vi "Main.vi"(7 "sweep rate, /min":dbl=0.2, 8 "sweep to:":dbl=-0.5, 9 "sweep":T6(radio)=enum."time_sweep") -> ()   [LabVIEW 2017] (continued)
                            n1353 = property on="data" class="Arr (strict)"("Value"=w1722) -> ()  [unwired: 2 in, 2 out]
                          }
                          frame #42 {
                            # "check if current \non 2461 SouceMeter\nis to be measured"
                            n1354 = property on="data" class="Arr (strict)"() -> ("Value"=w1730:dbl[])  [unwired: 2 in, 2 out]
                            n1355 = property on="iTC_Sample_T" class="Bool (strict)"() -> ("Value"=w1729:bool)  [unwired: 2 in, 2 out]
                            n1356 = case shown="True" w1729 {
                              tunnel: w1730 -> [w1732 w1737]
                              tunnel: [w1732 w1736] -> w1731
                              frame False {
                                # "we are not measuring 2461, voltage (2461_meas_v)"
                              }
                              frame True {
                                # "we are  measuring 2461, voltage (2461_meas_v)"
                                n1357 = property on="iTC_addr_sweep" class="VISAName"() -> ("Value"=w1735:refnum<visa-resource-name>)  [unwired: 2 in, 2 out]
                                n1358 = call "iTCread.vi"("VISA resource name"=w1735, "iTCreadCtrl"=iTCreadCtrl."Sample Temp") -> ("number"=w1733:dbl)  [unwired: 5 in, 3 out]
                                n1359 = Build Array (concatenate)(w1737, w1733) -> (w1736:dbl[])
                              }
                            }
                            n1360 = property on="data" class="Arr (strict)"("Value"=w1731) -> ()  [unwired: 2 in, 2 out]
                          }
                          frame #43 {
                            # "check if current \non 2461 SouceMeter\nis to be measured"
                            n1361 = property on="data" class="Arr (strict)"() -> ("Value"=w1739:dbl[])  [unwired: 2 in, 2 out]
                            n1362 = property on="VTI_T" class="Bool (strict)"() -> ("Value"=w1738:bool)  [unwired: 2 in, 2 out]
                            n1363 = case shown="True" w1738 {
                              tunnel: w1739 -> [w1741 w1746]
                              tunnel: [w1741 w1745] -> w1740
                              frame False {
                                # "we are not measuring 2461, voltage (2461_meas_v)"
                              }
                              frame True {
                                # "we are  measuring 2461, voltage (2461_meas_v)"
                                n1364 = property on="iTC_addr_sweep" class="VISAName"() -> ("Value"=w1744:refnum<visa-resource-name>)  [unwired: 2 in, 2 out]
                                n1365 = call "iTCread.vi"("VISA resource name"=w1744, "iTCreadCtrl"=iTCreadCtrl."VTI Temp") -> ("number"=w1742:dbl)  [unwired: 5 in, 3 out]
                                n1366 = Build Array (concatenate)(w1746, w1742) -> (w1745:dbl[])
                              }
                            }
                            n1367 = property on="data" class="Arr (strict)"("Value"=w1740) -> ()  [unwired: 2 in, 2 out]
                          }
                          frame #44 {
                            # "check if current \non 2461 SouceMeter\nis to be measured"
                            n1368 = property on="data" class="Arr (strict)"() -> ("Value"=w1748:dbl[])  [unwired: 2 in, 2 out]
                            n1369 = property on="PT1_T" class="Bool (strict)"() -> ("Value"=w1747:bool)  [unwired: 2 in, 2 out]
                            n1370 = case shown="True" w1747 {
                              tunnel: w1748 -> [w1750 w1755]
                              tunnel: [w1750 w1754] -> w1749
                              frame False {
                                # "we are not measuring 2461, voltage (2461_meas_v)"
                              }
                              frame True {
                                # "we are  measuring 2461, voltage (2461_meas_v)"
                                n1371 = property on="iTC_addr_sweep" class="VISAName"() -> ("Value"=w1753:refnum<visa-resource-name>)  [unwired: 2 in, 2 out]
                                n1372 = call "iTCread.vi"("VISA resource name"=w1753, "iTCreadCtrl"=iTCreadCtrl."PT1 Temp") -> ("number"=w1751:dbl)  [unwired: 5 in, 3 out]
                                n1373 = Build Array (concatenate)(w1755, w1751) -> (w1754:dbl[])
                              }
                            }
                            n1374 = property on="data" class="Arr (strict)"("Value"=w1749) -> ()  [unwired: 2 in, 2 out]
                          }
                          frame #45 {
                            # "check if current \non 2461 SouceMeter\nis to be measured"
                            n1375 = property on="data" class="Arr (strict)"() -> ("Value"=w1757:dbl[])  [unwired: 2 in, 2 out]
                            n1376 = property on="PT2_T" class="Bool (strict)"() -> ("Value"=w1756:bool)  [unwired: 2 in, 2 out]
                            n1377 = case shown="True" w1756 {
                              tunnel: w1757 -> [w1759 w1764]
                              tunnel: [w1759 w1763] -> w1758
                              frame False {
                                # "we are not measuring 2461, voltage (2461_meas_v)"
                              }
                              frame True {
                                # "we are  measuring 2461, voltage (2461_meas_v)"
                                n1378 = property on="iTC_addr_sweep" class="VISAName"() -> ("Value"=w1762:refnum<visa-resource-name>)  [unwired: 2 in, 2 out]
                                n1379 = call "iTCread.vi"("VISA resource name"=w1762, "iTCreadCtrl"=iTCreadCtrl."PT2 Temp") -> ("number"=w1760:dbl)  [unwired: 5 in, 3 out]
                                n1380 = Build Array (concatenate)(w1764, w1760) -> (w1763:dbl[])
                              }
                            }
                            n1381 = property on="data" class="Arr (strict)"("Value"=w1758) -> ()  [unwired: 2 in, 2 out]
                          }
                          frame #46 {
                            # "check if current \non 2461 SouceMeter\nis to be measured"
                            n1382 = property on="data" class="Arr (strict)"() -> ("Value"=w1766:dbl[])  [unwired: 2 in, 2 out]
                            n1383 = property on="VTI_P" class="Bool (strict)"() -> ("Value"=w1765:bool)  [unwired: 2 in, 2 out]
                            n1384 = case shown="True" w1765 {
                              tunnel: w1766 -> [w1768 w1773]
                              tunnel: [w1768 w1772] -> w1767
                              frame False {
                                # "we are not measuring 2461, voltage (2461_meas_v)"
                              }
                              frame True {
                                # "we are  measuring 2461, voltage (2461_meas_v)"
                                n1385 = property on="iTC_addr_sweep" class="VISAName"() -> ("Value"=w1771:refnum<visa-resource-name>)  [unwired: 2 in, 2 out]
                                n1386 = call "iTCread.vi"("VISA resource name"=w1771, "iTCreadCtrl"=iTCreadCtrl."VTI Pressure") -> ("number"=w1769:dbl)  [unwired: 5 in, 3 out]
                                n1387 = Build Array (concatenate)(w1773, w1769) -> (w1772:dbl[])
                              }
                            }
                            n1388 = property on="data" class="Arr (strict)"("Value"=w1767) -> ()  [unwired: 2 in, 2 out]
                          }
                          frame #47 {
                            # "check if current \non 2461 SouceMeter\nis to be measured"
                            n1389 = property on="2461_meas_v" class="Bool (strict)"() -> ("Value"=w1774:bool)  [unwired: 2 in, 2 out]
                            n1390 = property on="data" class="Arr (strict)"() -> ("Value"=w1775:dbl[])  [unwired: 2 in, 2 out]
                            n1391 = case shown="True" w1774 {
                              tunnel: w1775 -> [w1777 w1782]
                              tunnel: [w1777 w1781] -> w1776
                              frame False {
                                # "we are not measuring 2461, voltage (2461_meas_v)"
                              }
                              frame True {
                                # "we are  measuring 2461, voltage (2461_meas_v)"
                                n1392 = property on="2461_addr_sweep" class="VISAName"() -> ("Value"=w1779:refnum<visa-resource-name>)  [unwired: 2 in, 2 out]
                                n1393 = call <instrlib>:"Read (Single Point).vi"("VISA resource name"=w1779) -> ("Data out"=w1778:string)  [unwired: 12 in, 2 out]
                                n1394 = Fract/Exp String To Number(string=w1778) -> (number=w1780:dbl)  [unwired: 3 in, 1 out]
                                n1395 = Build Array (concatenate)(w1782, w1780) -> (w1781:dbl[])
                              }
                            }
                            n1396 = property on="data" class="Arr (strict)"("Value"=w1776) -> ()  [unwired: 2 in, 2 out]
                          }
                          frame #48 {
                            # "check if current \non 2461 SouceMeter\nis to be measured"
                            n1397 = property on="2461_meas_i" class="Bool (strict)"() -> ("Value"=w1783:bool)  [unwired: 2 in, 2 out]
                            n1398 = property on="data" class="Arr (strict)"() -> ("Value"=w1784:dbl[])  [unwired: 2 in, 2 out]
                            n1399 = case shown="True" w1783 {
                              tunnel: w1784 -> [w1786 w1790]
                              tunnel: [w1786 w1789] -> w1785
                              frame False {
                                # "we are not measuring 2461, voltage (2461_meas_v)"
                              }
                              frame True {
                                # "we are  measuring 2461, curent (2461_meas_i)"
                                n1400 = property on="2461_addr_sweep" class="VISAName"() -> ("Value"=w1788:refnum<visa-resource-name>)  [unwired: 2 in, 2 out]
                                n1401 = call <instrlib>:"Get Source Level.vi"("VISA resource name"=w1788) -> ("Current Level Out"=w1787:dbl)  [unwired: 7 in, 3 out]
                                n1402 = Build Array (concatenate)(w1790, w1787) -> (w1789:dbl[])
                              }
                            }
                            n1403 = property on="data" class="Arr (strict)"("Value"=w1785) -> ()  [unwired: 2 in, 2 out]
                          }
                        }
                      }
                    }
                  }
                }
              }
            }
          }
          frame #4 {
            n1404 = Enqueue Element(queue=w1791, element="Idle") -> ()  [unwired: 2 in, 3 out]
            n1405 = Wait (ms)(milliseconds to wait="Refresh Time(ms)") -> ()  [unwired: 1 out]
          }
        }
      }
      frame "Line Traces" {
      }
      frame "Start Sweep" {
        w1797 = dbl[][] []  # emty array for data
        # "0 = SR830_1_ip\n1 = SR830_1_oop\n2 = SR830_2_ip\n3 = SR830_2_oop\n4 = SR830_3_ip\n5 = SR830_3_oop\n6 = SR830_4_ip \n7 = SR830_4_oop \n8 = SR830_5_ip \n9 = SR830_5_oop \n10 = SR830_6_ip \n11 = SR830_6_oop\n12 = SR830_7_ip \n13 = SR830_7_oop\n14 = SR830_8_ip \n15 = SR830_8_oop\n16 = MFLI_V1\n17 = MFLI_I1\n18 = MFLI_V\n19 = MFLI_I\n20= 2400_1_v \n21= 2400_1_i \n22 = 2400_2_v\n23 = 2400_2_i \n24 = 2400_3_v \n25 = 2400_3_i \n26 = 2182A_1_ch1 \n27 = 2182A_1_ch2 \n28 = 2182A_2_ch1 \n29 = 2182A_2_ch2\n30 = 2182A_3_ch1 \n31 = 2182A_3_ch2 \n32 = 2182A_4_ch1 \n33 = 2182A_4_ch2 \n34 = 2636A_smua_v \n35 = 2636A_smua_i \n36 = 2636A_smub_v \n37 = 2636A_smub_i \n38 = time\n39 = iPS_Field\n40 = iPS_Magnet_T\n41 = iPS__SH_T\n42 = iTC _sample_T\n43 = iTC _VTI_T\n44 = iTC _PT1_T\n45 = iTC _PT2_T\n46 = iTC _VTI_P\n47 = 2461_meas_v\n48= 2461_meas_i\n49= Step_Value\n50= HyperLoop_Step\n51= SuperHyper_Step"
        # "initial time in seconds\nfrom the beginning of month"
        n1406 = stacked-sequence {
          tunnel: [_ _ w2676 _ _ _] -> w1794
          frame #0 {
            n1407 = local read "2636A smua meas v"() -> (w1804:bool)
            n1408 = local read "2636A smub meas v"() -> (w1802:bool)
            n1409 = local read "2636A smub meas i"() -> (w1801:bool)
            n1410 = local read "2636A smua meas i"() -> (w1803:bool)
            n1411 = property on="sweep" class="RadioBtnsControl (strict)"() -> ("Value"=w1799:T6)  [unwired: 2 in, 2 out]
            n1412 = Compound Arithmetic op=OR(w1804, w1803, w1802, w1801) -> (w1800:bool)
            n1413 = case shown="\"2461\"" w1799 {
              frame "2400_1" {
                # "add label for the first column in the datafile"
                n1414 = stacked-sequence {
                  frame #0 {
                    n1415 = property on="data_caption" class="Str"("Value"="") -> ()  [unwired: 2 in, 2 out]
                    n1416 = property on="Figure_axis" class="Arr (strict)"("Value"=string[] [] ("Figure_axis_string")) -> ()  [unwired: 2 in, 2 out]
                  }
                  frame #1 {
                    w1807 = "V_sweep_2400_1" ("V_sweep")
                    n1417 = Concatenate Strings(w1807, "\t") -> (w1809:string)
                    n1418 = Build Array(w1807) -> (w1808:string[])
                    n1419 = property on="data_caption" class="Str"("Value"=w1809) -> ()  [unwired: 2 in, 2 out]
                    n1420 = property on="Figure_axis" class="Arr (strict)"("Value"=w1808) -> ()  [unwired: 2 in, 2 out]
                  }
                }
              }
              frame "2400_2" {
                n1421 = stacked-sequence {
                  frame #0 {
                    n1422 = property on="data_caption" class="Str"("Value"="") -> ()  [unwired: 2 in, 2 out]
                    n1423 = property on="Figure_axis" class="Arr (strict)"("Value"=string[] [] ("Figure_axis_string")) -> ()  [unwired: 2 in, 2 out]
                  }
                  frame #1 {
                    w1813 = "V_sweep_2400_2" ("V_sweep")
                    n1424 = Build Array(w1813) -> (w1814:string[])
                    n1425 = Concatenate Strings(w1813, "\t") -> (w1816:string)
                    n1426 = property on="Figure_axis" class="Arr (strict)"("Value"=w1814) -> ()  [unwired: 2 in, 2 out]
                    n1427 = property on="data_caption" class="Str"("Value"=w1816) -> ()  [unwired: 2 in, 2 out]
                  }
                }
              }
              frame "2400_3" {
                n1428 = stacked-sequence {
                  frame #0 {
                    n1429 = property on="data_caption" class="Str"("Value"="") -> ()  [unwired: 2 in, 2 out]
                    n1430 = property on="Figure_axis" class="Arr (strict)"("Value"=string[] [] ("Figure_axis_string")) -> ()  [unwired: 2 in, 2 out]
                  }
                  frame #1 {
                    w1819 = "V_sweep_2400_3" ("V_sweep")
                    n1431 = Concatenate Strings(w1819, "\t") -> (w1822:string)
                    n1432 = Build Array(w1819) -> (w1820:string[])
                    n1433 = property on="data_caption" class="Str"("Value"=w1822) -> ()  [unwired: 2 in, 2 out]
                    n1434 = property on="Figure_axis" class="Arr (strict)"("Value"=w1820) -> ()  [unwired: 2 in, 2 out]
                  }
                }
              }
              frame "2636a_smua" {
                n1435 = stacked-sequence {
                  frame #0 {
                    n1436 = property on="data_caption" class="Str"("Value"="") -> ()  [unwired: 2 in, 2 out]
                    n1437 = property on="Figure_axis" class="Arr (strict)"("Value"=string[] [] ("Figure_axis_string")) -> ()  [unwired: 2 in, 2 out]
                  }
                  frame #1 {
                    w1825 = "V_sweep_2636a_smua" ("V_sweep")
                    n1438 = Concatenate Strings(w1825, "\t") -> (w1828:string)
                    n1439 = Build Array(w1825) -> (w1826:string[])
                    n1440 = property on="data_caption" class="Str"("Value"=w1828) -> ()  [unwired: 2 in, 2 out]
                    n1441 = property on="Figure_axis" class="Arr (strict)"("Value"=w1826) -> ()  [unwired: 2 in, 2 out]
                  }
                }
              }
              frame "2636a_smub" {
                n1442 = stacked-sequence {
                  frame #0 {
                    n1443 = property on="data_caption" class="Str"("Value"="") -> ()  [unwired: 2 in, 2 out]
                    n1444 = property on="Figure_axis" class="Arr (strict)"("Value"=string[] [] ("Figure_axis_string")) -> ()  [unwired: 2 in, 2 out]
                  }
                  frame #1 {
                    w1831 = "V_sweep_2636a_smub" ("V_sweep")
                    n1445 = Build Array(w1831) -> (w1832:string[])
                    n1446 = Concatenate Strings(w1831, "\t") -> (w1834:string)
                    n1447 = property on="Figure_axis" class="Arr (strict)"("Value"=w1832) -> ()  [unwired: 2 in, 2 out]
                    n1448 = property on="data_caption" class="Str"("Value"=w1834) -> ()  [unwired: 2 in, 2 out]
                  }
                }
              }
              frame "time_sweep", Default {
                n1449 = stacked-sequence {
                  frame #0 {
                    n1450 = property on="data_caption" class="Str"("Value"="") -> ()  [unwired: 2 in, 2 out]
                    n1451 = property on="Figure_axis" class="Arr (strict)"("Value"=string[] [] ("Figure_axis_string")) -> ()  [unwired: 2 in, 2 out]
                  }
                  frame #1 {
                    w1837 = "time_sweep" ("V_sweep")
                    n1452 = Build Array(w1837) -> (w1838:string[])
                    n1453 = Concatenate Strings(w1837, "\t") -> (w1839:string)
                    n1454 = property on="Figure_axis" class="Arr (strict)"("Value"=w1838) -> ()  [unwired: 2 in, 2 out]
                    n1455 = property on="data_caption" class="Str"("Value"=w1839) -> ()  [unwired: 2 in, 2 out]
                  }
                }
              }
              frame "iPS" {
                n1456 = stacked-sequence {
                  frame #0 {
                    n1457 = property on="data_caption" class="Str"("Value"="") -> ()  [unwired: 2 in, 2 out]
                    n1458 = property on="Figure_axis" class="Arr (strict)"("Value"=string[] [] ("Figure_axis_string")) -> ()  [unwired: 2 in, 2 out]
                  }
                  frame #1 {
                    w1843 = "Teslatron_iPS_OutputField" ("V_sweep")
                    n1459 = Build Array(w1843) -> (w1844:string[])
                    n1460 = Concatenate Strings(w1843, "\t") -> (w1846:string)
                    n1461 = property on="Figure_axis" class="Arr (strict)"("Value"=w1844) -> ()  [unwired: 2 in, 2 out]
                    n1462 = property on="data_caption" class="Str"("Value"=w1846) -> ()  [unwired: 2 in, 2 out]
                  }
                }
              }
              frame "iTC" {
                n1463 = stacked-sequence {
                  frame #0 {
                    n1464 = property on="data_caption" class="Str"("Value"="") -> ()  [unwired: 2 in, 2 out]
                    n1465 = property on="Figure_axis" class="Arr (strict)"("Value"=string[] ["", "SR830_1_ip", "SR830_1_oop", "SR830_2_ip", "SR830_2_oop", "2461_meas_v", "2461_meas_i", "2636A_smua_v", "2636A_smua_i", "formula"] ("Figure_axis")) -> ()  [unwired: 2 in, 2 out]
                  }
                  frame #1 {
                    w1851 = "Teslatron_iTC_Temp"
                    n1466 = Build Array(w1851) -> (w1850:string[])
                    n1467 = Concatenate Strings(w1851, "\t") -> (w1849:string)
                    n1468 = property on="data_caption" class="Str"("Value"=w1849) -> ()  [unwired: 2 in, 2 out]
                    n1469 = property on="Figure_axis" class="Arr (strict)"("Value"=w1850) -> ()  [unwired: 2 in, 2 out]
                  }
                }
              }
              frame "2461" {
                n1470 = stacked-sequence {
                  frame #0 {
                    n1471 = property on="data_caption" class="Str"("Value"="") -> ()  [unwired: 2 in, 2 out]
                    n1472 = property on="Figure_axis" class="Arr (strict)"("Value"=string[] ["", "SR830_1_ip", "SR830_1_oop", "SR830_2_ip", "SR830_2_oop", "2461_meas_v", "2461_meas_i", "2636A_smua_v", "2636A_smua_i", "formula"] ("Figure_axis")) -> ()  [unwired: 2 in, 2 out]
                  }
                  frame #1 {
                    w1857 = "I_sweep_2461"
                    n1473 = Build Array(w1857) -> (w1856:string[])
                    n1474 = Concatenate Strings(w1857, "\t") -> (w1855:string)
                    n1475 = property on="data_caption" class="Str"("Value"=w1855) -> ()  [unwired: 2 in, 2 out]
                    n1476 = property on="Figure_axis" class="Arr (strict)"("Value"=w1856) -> ()  [unwired: 2 in, 2 out]
                  }
                }
              }
            }
            n1477 = case shown="True" w1800 {
              frame False {
              }
              frame True {
                # "opens session for 2636a system sourcemeter"
                n1478 = local read "2336A addr"() -> (w1859:refnum<visa-resource-name>)
                n1479 = VISA Open(VISA resource name=w1859) -> ()  [unwired: 4 in, 2 out]
              }
            }
          }
          frame #1 {
            # "0 = SR830_1_ip\n1 = SR830_1_oop\n2 = SR830_2_ip\n3 = SR830_2_oop\n4 = SR830_3_ip\n5 = SR830_3_oop\n6 = SR830_4_ip \n7 = SR830_4_oop \n8 = SR830_5_ip \n9 = SR830_5_oop \n10 = SR830_6_ip \n11 = SR830_6_oop\n12 = SR830_7_ip \n13 = SR830_7_oop\n14 = SR830_8_ip \n15 = SR830_8_oop\n16 = MFLI_V1\n17 = MFLI_I1\n18 = MFLI_V2\n19 = MFLI_I2\n20= 2400_1_v \n21= 2400_1_i \n22 = 2400_2_v\n23 = 2400_2_i \n24 = 2400_3_v \n25 = 2400_3_i \n26 = 2182A_1_ch1 \n27 = 2182A_1_ch2 \n28 = 2182A_2_ch1 \n29 = 2182A_2_ch2\n30 = 2182A_3_ch1 \n31 = 2182A_3_ch2 \n32 = 2182A_4_ch1 \n33 = 2182A_4_ch2 \n34 = 2636A_smua_v \n35 = 2636A_smua_i \n36 = 2636A_smub_v \n37 = 2636A_smub_i \n38 = time\n39 = iPS_Field\n40 = iPS_Magnet_T\n41 = iPS__SH_T\n42 = iTC _sample_T\n43 = iTC _VTI_T\n44 = iTC _PT1_T\n45 = iTC _PT2_T\n46 = iTC _VTI_P\n47 = 2461_meas_v\n48= 2461_meas_i\n49= Step_Value\n50= HyperLoop_Step\n51= SuperHyper_Step"
            # "this part constructs the first (text) line for the data file with names of all measured variables,\nalso constructs a text array contaning names of all measured variable for the \"ring\" (so parameter can be selected and plotted)"
            n1480 = stacked-sequence {
              tunnel: [w1860 _ _ _ _ _ _ _ _ _ _ _ _ _ _ _ _ _ _ _ _ _ _ _ _ _ _ _ _ _ _ _ _ _ _ _ _ _ _ _ _ _ _ _ _ _ _ _ _ _ _ _] -> _
              frame #0 {
                # "SR830 1 in phase (SR830_1_ip)"
                n1481 = local read "SR830 1 ip"() -> (w1865:bool)
                n1482 = property on="Figure_axis" class="Arr (strict)"() -> ("Value"=w1862:string[])  [unwired: 2 in, 2 out]
                n1483 = property on="data_caption" class="Str"() -> ("Value"=w1864:string)  [unwired: 2 in, 2 out]
                n1484 = case shown="True" w1865 {
                  tunnel: w1864 -> [w1867 w1873]
                  tunnel: [w1867 w1872] -> w1863
                  tunnel: w1862 -> [w1866 w1870]
                  tunnel: [w1866 w1868] -> w1861
                  frame False {
                    # "not measure SR830 1 in phase signal (SR830_1_ip)"
                  }
                  frame True {
                    w1869 = "SR830_1_ip"
                    # "measure SR830 1 in phase signal (SR830_1_ip)"
                    n1485 = local read "SR830 1 addr"() -> (w1874:u8)
                    n1486 = Number To Decimal String(number=w1874) -> (decimal integer string=w1875:string)  [unwired: 1 in]
                    n1487 = GPIB Clear(3:w1875) -> ()  [unwired: 1 in, 2 out]
                    n1488 = Build Array (concatenate)(w1870, w1869) -> (w1868:string[])
                    n1489 = Concatenate Strings(w1873, w1869, "\t") -> (w1872:string)
                  }
                }
                n1490 = property on="Figure_axis" class="Arr (strict)"("Value"=w1861) -> ()  [unwired: 2 in, 2 out]
                n1491 = property on="data_caption" class="Str"("Value"=w1863) -> (error out=w1860:errorcluster)  [unwired: 2 in, 1 out]
              }
              frame #1 {
                # "SR830 1 out of phase (SR830_1_oop)"
                n1492 = local read "SR830 1 oop"() -> (w1880:bool)
                n1493 = property on="Figure_axis" class="Arr (strict)"() -> ("Value"=w1877:string[])  [unwired: 2 in, 2 out]
                n1494 = property on="data_caption" class="Str"() -> ("Value"=w1879:string)  [unwired: 2 in, 2 out]
                n1495 = case shown="False" w1880 {
                  tunnel: w1879 -> [w1882 w1888]
                  tunnel: [w1882 w1887] -> w1878
                  tunnel: w1877 -> [w1881 w1885]
                  tunnel: [w1881 w1883] -> w1876
                  frame False {
                    # "not measure SR830 1 out of phase signal (SR830_1_oop)"
                  }
                  frame True {
                    w1884 = "SR830_1_oop"
                    # "measure SR830 1 out of phase signal (SR830_1_oop)"
                    n1496 = local read "SR830 1 addr"() -> (w1889:u8)
                    n1497 = Number To Decimal String(number=w1889) -> (decimal integer string=w1890:string)  [unwired: 1 in]
                    n1498 = GPIB Clear(3:w1890) -> ()  [unwired: 1 in, 2 out]
                    n1499 = Build Array (concatenate)(w1885, w1884) -> (w1883:string[])
                    n1500 = Concatenate Strings(w1888, w1884, "\t") -> (w1887:string)
                  }
                }
                n1501 = property on="Figure_axis" class="Arr (strict)"("Value"=w1876) -> ()  [unwired: 2 in, 2 out]
                n1502 = property on="data_caption" class="Str"("Value"=w1878) -> ()  [unwired: 2 in, 2 out]
              }
              frame #2 {
                # "SR830 2 in phase (SR830_2_ip)"
                n1503 = local read "SR830 2 ip"() -> (w1895:bool)
                n1504 = property on="Figure_axis" class="Arr (strict)"() -> ("Value"=w1892:string[])  [unwired: 2 in, 2 out]
                n1505 = property on="data_caption" class="Str"() -> ("Value"=w1894:string)  [unwired: 2 in, 2 out]
                n1506 = case shown="True" w1895 {
                  tunnel: w1894 -> [w1897 w1903]
                  tunnel: [w1897 w1902] -> w1893
                  tunnel: w1892 -> [w1896 w1900]
                  tunnel: [w1896 w1898] -> w1891
                  frame False {
                    # "not measure SR830 2 in phase signal (SR830_2_ip)"
                  }
                  frame True {
                    w1899 = "SR830_2_ip"
                    # "measure SR830 2 in phase signal (SR830_2_ip)"
                    n1507 = local read "SR830 2 addr"() -> (w1904:u8)
                    n1508 = Number To Decimal String(number=w1904) -> (decimal integer string=w1905:string)  [unwired: 1 in]
                    n1509 = GPIB Clear(3:w1905) -> ()  [unwired: 1 in, 2 out]
                    n1510 = Build Array (concatenate)(w1900, w1899) -> (w1898:string[])
                    n1511 = Concatenate Strings(w1903, w1899, "\t") -> (w1902:string)
                  }
                }
                n1512 = property on="Figure_axis" class="Arr (strict)"("Value"=w1891) -> ()  [unwired: 2 in, 2 out]
                n1513 = property on="data_caption" class="Str"("Value"=w1893) -> ()  [unwired: 2 in, 2 out]
              }
              frame #3 {
                # "SR830 2 out of phase (SR830_2_oop)"
                n1514 = local read "SR830 2 oop"() -> (w1910:bool)
                n1515 = property on="Figure_axis" class="Arr (strict)"() -> ("Value"=w1907:string[])  [unwired: 2 in, 2 out]
                n1516 = property on="data_caption" class="Str"() -> ("Value"=w1909:string)  [unwired: 2 in, 2 out]
                n1517 = case shown="False" w1910 {
                  tunnel: w1909 -> [w1912 w1918]
                  tunnel: [w1912 w1917] -> w1908
                  tunnel: w1907 -> [w1911 w1915]
                  tunnel: [w1911 w1913] -> w1906
                  frame False {
                    # "not measure SR830 2 out of phase signal (SR830_2_oop)"
                  }
                  frame True {
                    w1914 = "SR830_2_oop"
                    # "measure SR830 2 out of phase signal (SR830_2_oop)"
                    n1518 = local read "SR830 2 addr"() -> (w1919:u8)
                    n1519 = Number To Decimal String(number=w1919) -> (decimal integer string=w1920:string)  [unwired: 1 in]
                    n1520 = GPIB Clear(3:w1920) -> ()  [unwired: 1 in, 2 out]
                    n1521 = Build Array (concatenate)(w1915, w1914) -> (w1913:string[])
                    n1522 = Concatenate Strings(w1918, w1914, "\t") -> (w1917:string)
                  }
                }
                n1523 = property on="Figure_axis" class="Arr (strict)"("Value"=w1906) -> ()  [unwired: 2 in, 2 out]
                n1524 = property on="data_caption" class="Str"("Value"=w1908) -> ()  [unwired: 2 in, 2 out]
              }
              frame #4 {
                # "SR830 3 in phase (SR830_3_ip)"
                n1525 = local read "SR830 3 ip"() -> (w1925:bool)
                n1526 = property on="Figure_axis" class="Arr (strict)"() -> ("Value"=w1922:string[])  [unwired: 2 in, 2 out]
                n1527 = property on="data_caption" class="Str"() -> ("Value"=w1924:string)  [unwired: 2 in, 2 out]
                n1528 = case shown="True" w1925 {
                  tunnel: w1924 -> [w1927 w1933]
                  tunnel: [w1927 w1932] -> w1923
                  tunnel: w1922 -> [w1926 w1930]
                  tunnel: [w1926 w1928] -> w1921
                  frame False {
                    # "not measure SR830 3 in phase signal (SR830_3_ip)"
                  }
                  frame True {
                    w1929 = "SR830_3_ip"
                    # "measure SR830 3 in phase signal (SR830_3_ip)"
                    n1529 = local read "SR830 3 addr"() -> (w1934:u8)
                    n1530 = Number To Decimal String(number=w1934) -> (decimal integer string=w1935:string)  [unwired: 1 in]
                    n1531 = GPIB Clear(3:w1935) -> ()  [unwired: 1 in, 2 out]
                    n1532 = Build Array (concatenate)(w1930, w1929) -> (w1928:string[])
                    n1533 = Concatenate Strings(w1933, w1929, "\t") -> (w1932:string)
                  }
                }
                n1534 = property on="Figure_axis" class="Arr (strict)"("Value"=w1921) -> ()  [unwired: 2 in, 2 out]
                n1535 = property on="data_caption" class="Str"("Value"=w1923) -> ()  [unwired: 2 in, 2 out]
              }
              frame #5 {
                # "SR830 3 out of phase (SR830_3_oop)"
                n1536 = local read "SR830 3 oop"() -> (w1940:bool)
                n1537 = property on="Figure_axis" class="Arr (strict)"() -> ("Value"=w1937:string[])  [unwired: 2 in, 2 out]
                n1538 = property on="data_caption" class="Str"() -> ("Value"=w1939:string)  [unwired: 2 in, 2 out]
                n1539 = case shown="True" w1940 {
                  tunnel: w1939 -> [w1942 w1948]
                  tunnel: [w1942 w1947] -> w1938
                  tunnel: w1937 -> [w1941 w1945]
                  tunnel: [w1941 w1943] -> w1936
                  frame False {
                    # "not measure SR830 3 out of phase signal (SR830_3_oop)"
                  }
                  frame True {
                    w1944 = "SR830_3_oop"
                    # "measure SR830 3 out phase signal (SR830_3_oop)"
                    n1540 = local read "SR830 3 addr"() -> (w1949:u8)
                    n1541 = Number To Decimal String(number=w1949) -> (decimal integer string=w1950:string)  [unwired: 1 in]
                    n1542 = GPIB Clear(3:w1950) -> ()  [unwired: 1 in, 2 out]
                    n1543 = Build Array (concatenate)(w1945, w1944) -> (w1943:string[])
                    n1544 = Concatenate Strings(w1948, w1944, "\t") -> (w1947:string)
                  }
                }
                n1545 = property on="Figure_axis" class="Arr (strict)"("Value"=w1936) -> ()  [unwired: 2 in, 2 out]
                n1546 = property on="data_caption" class="Str"("Value"=w1938) -> ()  [unwired: 2 in, 2 out]
              }
              frame #6 {
                # "SR830 4 in phase (SR830_4_ip)"
                n1547 = local read "SR830 4 ip"() -> (w1955:bool)
                n1548 = property on="Figure_axis" class="Arr (strict)"() -> ("Value"=w1952:string[])  [unwired: 2 in, 2 out]
                n1549 = property on="data_caption" class="Str"() -> ("Value"=w1954:string)  [unwired: 2 in, 2 out]
                n1550 = case shown="False" w1955 {
                  tunnel: w1954 -> [w1957 w1963]
                  tunnel: [w1957 w1962] -> w1953
                  tunnel: w1952 -> [w1956 w1960]
                  tunnel: [w1956 w1958] -> w1951
                  frame False {
                    # "not measure SR830 4 in phase signal (SR830_4_ip)"
                  }
                  frame True {
                    w1959 = "SR830_4_ip"
                    # "measure SR830 4 in phase signal (SR830_4_ip)"
                    n1551 = local read "SR830 4 addr"() -> (w1964:u8)
                    n1552 = Number To Decimal String(number=w1964) -> (decimal integer string=w1965:string)  [unwired: 1 in]
                    n1553 = GPIB Clear(3:w1965) -> ()  [unwired: 1 in, 2 out]
                    n1554 = Build Array (concatenate)(w1960, w1959) -> (w1958:string[])
                    n1555 = Concatenate Strings(w1963, w1959, "\t") -> (w1962:string)
                  }
                }
                n1556 = property on="Figure_axis" class="Arr (strict)"("Value"=w1951) -> ()  [unwired: 2 in, 2 out]
                n1557 = property on="data_caption" class="Str"("Value"=w1953) -> ()  [unwired: 2 in, 2 out]
              }
              frame #7 {
                # "SR830 4 out of phase (SR830_4_oop)"
                n1558 = local read "SR830 4 oop"() -> (w1970:bool)
                n1559 = property on="Figure_axis" class="Arr (strict)"() -> ("Value"=w1967:string[])  [unwired: 2 in, 2 out]
                n1560 = property on="data_caption" class="Str"() -> ("Value"=w1969:string)  [unwired: 2 in, 2 out]
                n1561 = case shown="False" w1970 {
                  tunnel: w1969 -> [w1972 w1978]
                  tunnel: [w1972 w1977] -> w1968
                  tunnel: w1967 -> [w1971 w1975]
                  tunnel: [w1971 w1973] -> w1966
                  frame False {
                    # "not measure SR830 4 out of phase signal (SR830_4_oop)"
                  }
                  frame True {
                    w1974 = "SR830_4_oop"
                    # "measure SR830 4 out of phase signal (SR830_4_oop)"
                    n1562 = local read "SR830 4 addr"() -> (w1979:u8)
                    n1563 = Number To Decimal String(number=w1979) -> (decimal integer string=w1980:string)  [unwired: 1 in]
                    n1564 = GPIB Clear(3:w1980) -> ()  [unwired: 1 in, 2 out]
                    n1565 = Build Array (concatenate)(w1975, w1974) -> (w1973:string[])
                    n1566 = Concatenate Strings(w1978, w1974, "\t") -> (w1977:string)
                  }
                }
                n1567 = property on="Figure_axis" class="Arr (strict)"("Value"=w1966) -> ()  [unwired: 2 in, 2 out]
                n1568 = property on="data_caption" class="Str"("Value"=w1968) -> ()  [unwired: 2 in, 2 out]
              }
              frame #8 {
                # "SR830 5 in phase (SR830_5_ip)"
                n1569 = local read "SR830 5 ip"() -> (w1985:bool)
                n1570 = property on="Figure_axis" class="Arr (strict)"() -> ("Value"=w1982:string[])  [unwired: 2 in, 2 out]
                n1571 = property on="data_caption" class="Str"() -> ("Value"=w1984:string)  [unwired: 2 in, 2 out]
                n1572 = case shown="True" w1985 {
                  tunnel: w1984 -> [w1987 w1993]
                  tunnel: [w1987 w1992] -> w1983
                  tunnel: w1982 -> [w1986 w1990]
                  tunnel: [w1986 w1988] -> w1981
                  frame False {
                    # "not measure SR830 5 in phase signal (SR830_5_ip)"
                  }
                  frame True {
                    w1989 = "SR830_5_ip"
                    # "measure SR830 5 in phase signal (SR830_5_ip)"
                    n1573 = local read "SR830 5 addr"() -> (w1994:u8)
                    n1574 = Number To Decimal String(number=w1994) -> (decimal integer string=w1995:string)  [unwired: 1 in]
                    n1575 = GPIB Clear(3:w1995) -> ()  [unwired: 1 in, 2 out]
                    n1576 = Build Array (concatenate)(w1990, w1989) -> (w1988:string[])
                    n1577 = Concatenate Strings(w1993, w1989, "\t") -> (w1992:string)
                  }
                }
                n1578 = property on="Figure_axis" class="Arr (strict)"("Value"=w1981) -> ()  [unwired: 2 in, 2 out]
                n1579 = property on="data_caption" class="Str"("Value"=w1983) -> ()  [unwired: 2 in, 2 out]
              }
              frame #9 {
                # "SR830 5 out of phase (SR830_5_oop)"
                n1580 = local read "SR830 5 oop"() -> (w2000:bool)
                n1581 = property on="Figure_axis" class="Arr (strict)"() -> ("Value"=w1997:string[])  [unwired: 2 in, 2 out]
                n1582 = property on="data_caption" class="Str"() -> ("Value"=w1999:string)  [unwired: 2 in, 2 out]
                n1583 = case shown="True" w2000 {
                  tunnel: w1999 -> [w2002 w2008]
                  tunnel: [w2002 w2007] -> w1998
                  tunnel: w1997 -> [w2001 w2005]
                  tunnel: [w2001 w2003] -> w1996
                  frame False {
                    # "not measure SR830 5 out of phase signal (SR830_5_oop)"
                  }
                  frame True {
                    w2004 = "SR830_5_oop"
                    # "measure SR830 5 out of phase signal (SR830_5_oop)"
                    n1584 = local read "SR830 5 addr"() -> (w2009:u8)
                    n1585 = Number To Decimal String(number=w2009) -> (decimal integer string=w2010:string)  [unwired: 1 in]
                    n1586 = GPIB Clear(3:w2010) -> ()  [unwired: 1 in, 2 out]
                    n1587 = Build Array (concatenate)(w2005, w2004) -> (w2003:string[])
                    n1588 = Concatenate Strings(w2008, w2004, "\t") -> (w2007:string)
                  }
                }
                n1589 = property on="Figure_axis" class="Arr (strict)"("Value"=w1996) -> ()  [unwired: 2 in, 2 out]
                n1590 = property on="data_caption" class="Str"("Value"=w1998) -> ()  [unwired: 2 in, 2 out]
              }
              frame #10 {
                # "SR830 6 in phase (SR830_6_ip)"
                n1591 = property on="SR830_6_ip" class="Bool (strict)"() -> ("Value"=w2011:bool)  [unwired: 2 in, 2 out]
                n1592 = property on="Figure_axis" class="Arr (strict)"() -> ("Value"=w2013:string[])  [unwired: 2 in, 2 out]
                n1593 = property on="data_caption" class="Str"() -> ("Value"=w2015:string)  [unwired: 2 in, 2 out]
                n1594 = case shown="True" w2011 {
                  tunnel: w2015 -> [w2017 w2023]
                  tunnel: [w2017 w2022] -> w2014
                  tunnel: w2013 -> [w2016 w2020]
                  tunnel: [w2016 w2018] -> w2012
                  frame False {
                    # "not measure SR830 6 in phase signal (SR830_6_ip)"
                  }
                  frame True {
                    w2019 = "SR830_6_ip"
                    # "measure SR830 6 in phase signal (SR830_6_ip)"
                    n1595 = local read "SR830_6"() -> (w2024:u8)
                    n1596 = Number To Decimal String(number=w2024) -> (decimal integer string=w2025:string)  [unwired: 1 in]
                    n1597 = GPIB Clear(3:w2025) -> ()  [unwired: 1 in, 2 out]
                    n1598 = Build Array (concatenate)(w2020, w2019) -> (w2018:string[])
                    n1599 = Concatenate Strings(w2023, w2019, "\t") -> (w2022:string)
                  }
                }
                n1600 = property on="Figure_axis" class="Arr (strict)"("Value"=w2012) -> ()  [unwired: 2 in, 2 out]
                n1601 = property on="data_caption" class="Str"("Value"=w2014) -> ()  [unwired: 2 in, 2 out]
              }
              frame #11 {
                # "SR830 6 out of phase (SR830_6_oop)"
                n1602 = local read "SR830_6_oop"() -> (w2030:bool)
                n1603 = property on="Figure_axis" class="Arr (strict)"() -> ("Value"=w2027:string[])  [unwired: 2 in, 2 out]
                n1604 = property on="data_caption" class="Str"() -> ("Value"=w2029:string)  [unwired: 2 in, 2 out]
                n1605 = case shown="False" w2030 {
                  tunnel: w2029 -> [w2032 w2038]
                  tunnel: [w2032 w2037] -> w2028
                  tunnel: w2027 -> [w2031 w2035]
                  tunnel: [w2031 w2033] -> w2026
                  frame False {
                    # "not measure SR830 6 out of phase signal (SR830_6_oop)"
                  }
                  frame True {
                    w2034 = "SR830_6_oop"
                    # "measure SR830 6 out of phase signal (SR830_6_oop)"
                    n1606 = local read "SR830_6"() -> (w2039:u8)
                    n1607 = Number To Decimal String(number=w2039) -> (decimal integer string=w2040:string)  [unwired: 1 in]
                    n1608 = GPIB Clear(3:w2040) -> ()  [unwired: 1 in, 2 out]
                    n1609 = Build Array (concatenate)(w2035, w2034) -> (w2033:string[])
                    n1610 = Concatenate Strings(w2038, w2034, "\t") -> (w2037:string)
                  }
                }
                n1611 = property on="Figure_axis" class="Arr (strict)"("Value"=w2026) -> ()  [unwired: 2 in, 2 out]
                n1612 = property on="data_caption" class="Str"("Value"=w2028) -> ()  [unwired: 2 in, 2 out]
              }
              frame #12 {
                # "SR830 7 in phase (SR830_7_ip)"
                n1613 = local read "SR830_7_ip"() -> (w2041:bool)
                n1614 = property on="Figure_axis" class="Arr (strict)"() -> ("Value"=w2043:string[])  [unwired: 2 in, 2 out]
                n1615 = property on="data_caption" class="Str"() -> ("Value"=w2045:string)  [unwired: 2 in, 2 out]
                n1616 = case shown="True" w2041 {
                  tunnel: w2045 -> [w2047 w2053]
                  tunnel: [w2047 w2052] -> w2044
                  tunnel: w2043 -> [w2046 w2050]
                  tunnel: [w2046 w2048] -> w2042
                  frame False {
                    # "not measure SR830 7 in phase signal (SR830_7_ip)"
                  }
                  frame True {
                    w2049 = "SR830_7_ip"
                    # "measure SR830 7 in phase signal (SR830_7_ip)"
                    n1617 = local read "SR830_7"() -> (w2054:u8)
                    n1618 = Number To Decimal String(number=w2054) -> (decimal integer string=w2055:string)  [unwired: 1 in]
                    n1619 = GPIB Clear(3:w2055) -> ()  [unwired: 1 in, 2 out]
                    n1620 = Build Array (concatenate)(w2050, w2049) -> (w2048:string[])
                    n1621 = Concatenate Strings(w2053, w2049, "\t") -> (w2052:string)
                  }
                }
                n1622 = property on="Figure_axis" class="Arr (strict)"("Value"=w2042) -> ()  [unwired: 2 in, 2 out]
                n1623 = property on="data_caption" class="Str"("Value"=w2044) -> ()  [unwired: 2 in, 2 out]
              }
              frame #13 {
                # "SR830 7 out of phase (SR830_7_oop)"
                n1624 = local read "SR830_7_oop"() -> (w2060:bool)
                n1625 = property on="Figure_axis" class="Arr (strict)"() -> ("Value"=w2057:string[])  [unwired: 2 in, 2 out]
                n1626 = property on="data_caption" class="Str"() -> ("Value"=w2059:string)  [unwired: 2 in, 2 out]
                n1627 = case shown="True" w2060 {
                  tunnel: w2059 -> [w2062 w2068]
                  tunnel: [w2062 w2067] -> w2058
                  tunnel: w2057 -> [w2061 w2065]
                  tunnel: [w2061 w2063] -> w2056
                  frame False {
                    # "not measure SR830 7 out of phase signal (SR830_7_oop)"
                  }
                  frame True {
                    w2064 = "SR830_7_oop"
                    # "measure SR830 7 out of phase signal (SR830_7_oop)"
                    n1628 = local read "SR830_7"() -> (w2069:u8)
                    n1629 = Number To Decimal String(number=w2069) -> (decimal integer string=w2070:string)  [unwired: 1 in]
                    n1630 = GPIB Clear(3:w2070) -> ()  [unwired: 1 in, 2 out]
                    n1631 = Build Array (concatenate)(w2065, w2064) -> (w2063:string[])
                    n1632 = Concatenate Strings(w2068, w2064, "\t") -> (w2067:string)
                  }
                }
                n1633 = property on="Figure_axis" class="Arr (strict)"("Value"=w2056) -> ()  [unwired: 2 in, 2 out]
                n1634 = property on="data_caption" class="Str"("Value"=w2058) -> ()  [unwired: 2 in, 2 out]
              }
              frame #14 {
                # "SR830 8 in phase (SR830_8_ip)"
                n1635 = local read "SR830_8_ip"() -> (w2071:bool)
                n1636 = property on="Figure_axis" class="Arr (strict)"() -> ("Value"=w2073:string[])  [unwired: 2 in, 2 out]
                n1637 = property on="data_caption" class="Str"() -> ("Value"=w2075:string)  [unwired: 2 in, 2 out]
                n1638 = case shown="True" w2071 {
                  tunnel: w2075 -> [w2077 w2083]
                  tunnel: [w2077 w2082] -> w2074
                  tunnel: w2073 -> [w2076 w2080]
                  tunnel: [w2076 w2078] -> w2072
                  frame False {
                    # "not measure SR830 8 in phase signal (SR830_8_ip)"
                  }
                  frame True {
                    w2079 = "SR830_8_ip"
                    # "measure SR830 8 in phase signal (SR830_8_ip)"
                    n1639 = local read "SR830_8"() -> (w2084:u8)
                    n1640 = Number To Decimal String(number=w2084) -> (decimal integer string=w2085:string)  [unwired: 1 in]
                    n1641 = GPIB Clear(3:w2085) -> ()  [unwired: 1 in, 2 out]
                    n1642 = Build Array (concatenate)(w2080, w2079) -> (w2078:string[])
                    n1643 = Concatenate Strings(w2083, w2079, "\t") -> (w2082:string)
                  }
                }
                n1644 = property on="Figure_axis" class="Arr (strict)"("Value"=w2072) -> ()  [unwired: 2 in, 2 out]
                n1645 = property on="data_caption" class="Str"("Value"=w2074) -> ()  [unwired: 2 in, 2 out]
              }
              frame #15 {
                # "SR830 8 out phase (SR830_8_oop)"
                n1646 = local read "SR830_8_oop"() -> (w2086:bool)
                n1647 = property on="Figure_axis" class="Arr (strict)"() -> ("Value"=w2088:string[])  [unwired: 2 in, 2 out]
                n1648 = property on="data_caption" class="Str"() -> ("Value"=w2090:string)  [unwired: 2 in, 2 out]
                n1649 = case shown="True" w2086 {
                  tunnel: w2090 -> [w2092 w2098]
                  tunnel: [w2092 w2097] -> w2089
                  tunnel: w2088 -> [w2091 w2095]
                  tunnel: [w2091 w2093] -> w2087
                  frame False {
                    # "not measure SR830 8 out phase signal (SR830_8_oop)"
                  }
                  frame True {
                    w2094 = "SR830_8_oop"
                    # "measure SR830 8 out phase signal (SR830_8_00p)"
                    n1650 = local read "SR830_8"() -> (w2099:u8)
                    n1651 = Number To Decimal String(number=w2099) -> (decimal integer string=w2100:string)  [unwired: 1 in]
                    n1652 = GPIB Clear(3:w2100) -> ()  [unwired: 1 in, 2 out]
                    n1653 = Build Array (concatenate)(w2095, w2094) -> (w2093:string[])
                    n1654 = Concatenate Strings(w2098, w2094, "\t") -> (w2097:string)
                  }
                }
                n1655 = property on="Figure_axis" class="Arr (strict)"("Value"=w2087) -> ()  [unwired: 2 in, 2 out]
                n1656 = property on="data_caption" class="Str"("Value"=w2089) -> ()  [unwired: 2 in, 2 out]
              }
              frame #16 {
                # "MFLI_V1"
                n1657 = property on="MFLI_1" class="Str" props=["Value"]() -> ()  [unwired: 2 in, 3 out]
                n1658 = property on="MFLI_V1" class="Bool (strict)"() -> ("Value"=w2101:bool)  [unwired: 2 in, 2 out]
                n1659 = property on="data_caption" class="Str"() -> ("Value"=w2105:string)  [unwired: 2 in, 2 out]
                n1660 = property on="Figure_axis" class="Arr (strict)"() -> ("Value"=w2103:string[])  [unwired: 2 in, 2 out]
                n1661 = case shown="True" w2101 {
                  tunnel: w2105 -> [w2107 w2117]
                  tunnel: [w2107 w2116] -> w2104
                  tunnel: w2103 -> [w2106 w2115]
                  tunnel: [w2106 w2114] -> w2102
                  frame False {
                    # "not measure 2461 voltage (2461_meas_v)"
                  }
                  frame True {
                    w2112 = "MFLI_Vy_1"
                    w2113 = "MFLI_Vx_1"
                    w2111 = "\t"
                    w2110 = "MFLI_freq_1"
                    n1662 = property on="HandleOut" class="Clust (strict)"() -> ("Value"=w2109:T5)  [unwired: 2 in, 2 out]
                    n1663 = Unbundle(w2109) -> ("Connected"=w2108:bool)  [unwired: 5 out]
                    n1664 = case shown="False" w2108 {
                      frame False {
                        n1665 = property on="MFLI_1" class="Str"() -> ("Value"=w2120:string)  [unwired: 2 in, 2 out]
                        n1666 = call <instrlib>:"ziOpen.vi"("Address"=w2120) -> ("HandleOut"=w2119:T5)  [unwired: 3 in, 2 out]
                        n1667 = call <instrlib>:"ziCheckVersion.vi"("Handle In"=w2119) -> ("Handle Out"=w2118:T5)  [unwired: 12 in, 2 out]
                        n1668 = property on="HandleOut" class="Clust (strict)"("Value"=w2118) -> ()  [unwired: 2 in, 2 out]
                      }
                      frame True {
                      }
                    }
                    n1669 = Build Array (concatenate)(w2115, w2113, w2112, w2110) -> (w2114:string[])
                    n1670 = Concatenate Strings(w2117, w2113, w2111, w2112, w2111, w2110, w2111) -> (w2116:string)
                  }
                }
                n1671 = property on="Figure_axis" class="Arr (strict)"("Value"=w2102) -> ()  [unwired: 2 in, 2 out]
                n1672 = property on="data_caption" class="Str"("Value"=w2104) -> ()  [unwired: 2 in, 2 out]
              }
              frame #17 {
                # "MFLI_I1"
                n1673 = property on="MFLI_I1" class="Bool (strict)"() -> ("Value"=w2121:bool)  [unwired: 2 in, 2 out]
                n1674 = property on="data_caption" class="Str"() -> ("Value"=w2125:string)  [unwired: 2 in, 2 out]
                n1675 = property on="Figure_axis" class="Arr (strict)"() -> ("Value"=w2123:string[])  [unwired: 2 in, 2 out]
                n1676 = case shown="True" w2121 {
                  tunnel: w2125 -> [w2127 w2137]
                  tunnel: [w2127 w2136] -> w2124
                  tunnel: w2123 -> [w2126 w2135]
                  tunnel: [w2126 w2134] -> w2122
                  frame False {
                    # "not measure 2461 voltage (2461_meas_v)"
                  }
                  frame True {
                    w2132 = "MFLI_Iy-1"
                    w2133 = "MFLI_Ix_1"
                    w2131 = "\t"
                    w2130 = "MFLI_freq_1"
                    n1677 = property on="HandleOut" class="Clust (strict)"() -> ("Value"=w2129:T5)  [unwired: 2 in, 2 out]
                    n1678 = Unbundle(w2129) -> ("Connected"=w2128:bool)  [unwired: 5 out]
                    n1679 = case shown="False" w2128 {
                      frame False {
                        n1680 = property on="MFLI_1" class="Str"() -> ("Value"=w2140:string)  [unwired: 2 in, 2 out]
                        n1681 = call <instrlib>:"ziOpen.vi"("Address"=w2140) -> ("HandleOut"=w2139:T5)  [unwired: 3 in, 2 out]
                        n1682 = call <instrlib>:"ziCheckVersion.vi"("Handle In"=w2139) -> ("Handle Out"=w2138:T5)  [unwired: 12 in, 2 out]
                        n1683 = property on="HandleOut" class="Clust (strict)"("Value"=w2138) -> ()  [unwired: 2 in, 2 out]
                      }
                      frame True {
                      }
                    }
                    n1684 = Build Array (concatenate)(w2135, w2133, w2132, w2130) -> (w2134:string[])
                    n1685 = Concatenate Strings(w2137, w2133, w2131, w2132, w2131, w2130, w2131) -> (w2136:string)
                  }
                }
                n1686 = property on="Figure_axis" class="Arr (strict)"("Value"=w2122) -> ()  [unwired: 2 in, 2 out]
                n1687 = property on="data_caption" class="Str"("Value"=w2124) -> ()  [unwired: 2 in, 2 out]
              }
              frame #18 {
                # "MFLI_V 2"
                n1688 = local read "MFLI_V2"() -> (w2141:bool)
                n1689 = property on="data_caption" class="Str"() -> ("Value"=w2145:string)  [unwired: 2 in, 2 out]
                n1690 = property on="Figure_axis" class="Arr (strict)"() -> ("Value"=w2143:string[])  [unwired: 2 in, 2 out]
                n1691 = case shown="True" w2141 {
                  tunnel: w2145 -> [w2147 w2157]
                  tunnel: [w2147 w2156] -> w2144
                  tunnel: w2143 -> [w2146 w2155]
                  tunnel: [w2146 w2154] -> w2142
                  frame False {
                  }
                  frame True {
                    w2152 = "MFLI_Vy_2"
                    w2153 = "MFLI_Vx_2"
                    w2151 = "\t"
                    w2150 = "MFLI_freq_2"
                    n1692 = property on="Handle Out 2" class="Clust (strict)"() -> ("Value"=w2149:T5)  [unwired: 2 in, 2 out]
                    n1693 = Unbundle(w2149) -> ("Connected"=w2148:bool)  [unwired: 5 out]
                    n1694 = case shown="False" w2148 {
                      frame False {
                        n1695 = local read "MFLI_2"() -> (w2158:string)
                        n1696 = call <instrlib>:"ziOpen.vi"("Address"=w2158) -> ("HandleOut"=w2160:T5)  [unwired: 3 in, 2 out]
                        n1697 = call <instrlib>:"ziCheckVersion.vi"("Handle In"=w2160) -> ("Handle Out"=w2159:T5)  [unwired: 12 in, 2 out]
                        n1698 = property on="Handle Out 2" class="Clust (strict)"("Value"=w2159) -> ()  [unwired: 2 in, 2 out]
                      }
                      frame True {
                      }
                    }
                    n1699 = Build Array (concatenate)(w2155, w2153, w2152, w2150) -> (w2154:string[])
                    n1700 = Concatenate Strings(w2157, w2153, w2151, w2152, w2151, w2150, w2151) -> (w2156:string)
                  }
                }
                n1701 = property on="Figure_axis" class="Arr (strict)"("Value"=w2142) -> ()  [unwired: 2 in, 2 out]
                n1702 = property on="data_caption" class="Str"("Value"=w2144) -> ()  [unwired: 2 in, 2 out]
              }
              frame #19 {
                # "MFLI_I 2"
                n1703 = local read "MFLI_I2"() -> (w2161:bool)
                n1704 = property on="data_caption" class="Str"() -> ("Value"=w2165:string)  [unwired: 2 in, 2 out]
                n1705 = property on="Figure_axis" class="Arr (strict)"() -> ("Value"=w2163:string[])  [unwired: 2 in, 2 out]
                n1706 = case shown="True" w2161 {
                  tunnel: w2165 -> [w2167 w2177]
                  tunnel: [w2167 w2176] -> w2164
                  tunnel: w2163 -> [w2166 w2175]
                  tunnel: [w2166 w2174] -> w2162
                  frame False {
                    # "not measure 2461 voltage (2461_meas_v)"
                  }
                  frame True {
                    w2172 = "MFLI_Iy_2"
                    w2173 = "MFLI_Ix_2"
                    w2171 = "\t"
                    w2170 = "MFLI_freq_2"
                    n1707 = property on="Handle Out 2" class="Clust (strict)"() -> ("Value"=w2169:T5)  [unwired: 2 in, 2 out]
                    n1708 = Unbundle(w2169) -> ("Connected"=w2168:bool)  [unwired: 5 out]
                    n1709 = case shown="False" w2168 {
                      frame False {
                        n1710 = local read "MFLI_2"() -> (w2178:string)
                        n1711 = call <instrlib>:"ziOpen.vi"("Address"=w2178) -> ("HandleOut"=w2180:T5)  [unwired: 3 in, 2 out]
                        n1712 = call <instrlib>:"ziCheckVersion.vi"("Handle In"=w2180) -> ("Handle Out"=w2179:T5)  [unwired: 12 in, 2 out]
                        n1713 = property on="Handle Out 2" class="Clust (strict)"("Value"=w2179) -> ()  [unwired: 2 in, 2 out]
                      }
                      frame True {
                      }
                    }
                    n1714 = Build Array (concatenate)(w2175, w2173, w2172, w2170) -> (w2174:string[])
                    n1715 = Concatenate Strings(w2177, w2173, w2171, w2172, w2171, w2170, w2171) -> (w2176:string)
                  }
                }
                n1716 = property on="Figure_axis" class="Arr (strict)"("Value"=w2162) -> ()  [unwired: 2 in, 2 out]
                n1717 = property on="data_caption" class="Str"("Value"=w2164) -> ()  [unwired: 2 in, 2 out]
              }
              frame #20 {
                # "2400 1 voltage measure (2400_1_v)"
                n1718 = local read "2400 1 meas v"() -> (w2185:bool)
                n1719 = property on="Figure_axis" class="Arr (strict)"() -> ("Value"=w2182:string[])  [unwired: 2 in, 2 out]
                n1720 = property on="data_caption" class="Str"() -> ("Value"=w2184:string)  [unwired: 2 in, 2 out]
                n1721 = case shown="False" w2185 {
                  tunnel: w2184 -> [w2187 w2193]
                  tunnel: [w2187 w2192] -> w2183
                  tunnel: w2182 -> [w2186 w2190]
                  tunnel: [w2186 w2188] -> w2181
                  frame False {
                    # "not measure 2400 1 voltage (2400_1_v)"
                  }
                  frame True {
                    w2189 = "2400_1_v"
                    # "measure 2400 1 voltage (2400_1_v)"
                    n1722 = local read "2400 1 addr"() -> (w2194:u8)
                    n1723 = Number To Decimal String(number=w2194) -> (decimal integer string=w2195:string)  [unwired: 1 in]
                    n1724 = GPIB Clear(3:w2195) -> ()  [unwired: 1 in, 2 out]
                    n1725 = Build Array (concatenate)(w2190, w2189) -> (w2188:string[])
                    n1726 = Concatenate Strings(w2193, w2189, "\t") -> (w2192:string)
                  }
                }
                n1727 = property on="Figure_axis" class="Arr (strict)"("Value"=w2181) -> ()  [unwired: 2 in, 2 out]
                n1728 = property on="data_caption" class="Str"("Value"=w2183) -> ()  [unwired: 2 in, 2 out]
              }
              frame #21 {
                # "2400 1 current measure (2400_1_i)"
                n1729 = local read "2400 1 meas i"() -> (w2200:bool)
                n1730 = property on="Figure_axis" class="Arr (strict)"() -> ("Value"=w2197:string[])  [unwired: 2 in, 2 out]
                n1731 = property on="data_caption" class="Str"() -> ("Value"=w2199:string)  [unwired: 2 in, 2 out]
                n1732 = case shown="False" w2200 {
                  tunnel: w2199 -> [w2202 w2208]
                  tunnel: [w2202 w2207] -> w2198
